vi "StartAndorCamera.vi"(2 "error in (no error)":errorcluster, 3 "Initial temp":i32) -> (0 "error out":errorcluster, 1 "Camera OK?":bool)   [LabVIEW 2019]
uses:
  <userlib>/atmcd32d.llb/Shutter_type typedef.ctl
  <userlib>/atmcd32d.llb/Shutter_mode typedef.ctl
panel:
  out "DLL error code":u32
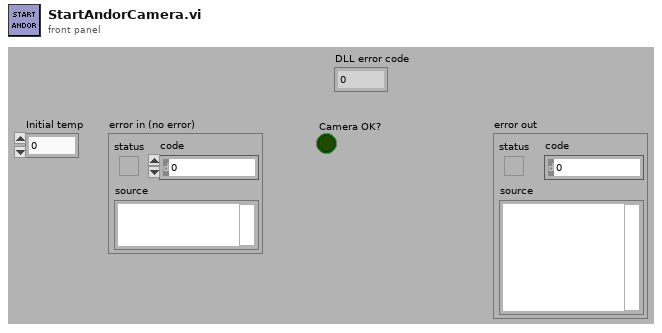
[diagram p1: front panel]
types:
  T1 = typedef "Shutter_mode typedef.ctl" = enum16{"Auto", "Open", "Close", "N/A (3)", "Open FVB Series", "Open Any Series"}
  T2 = typedef "Shutter_type typedef.ctl" = enum16{"TTL Low", "TTL High"}
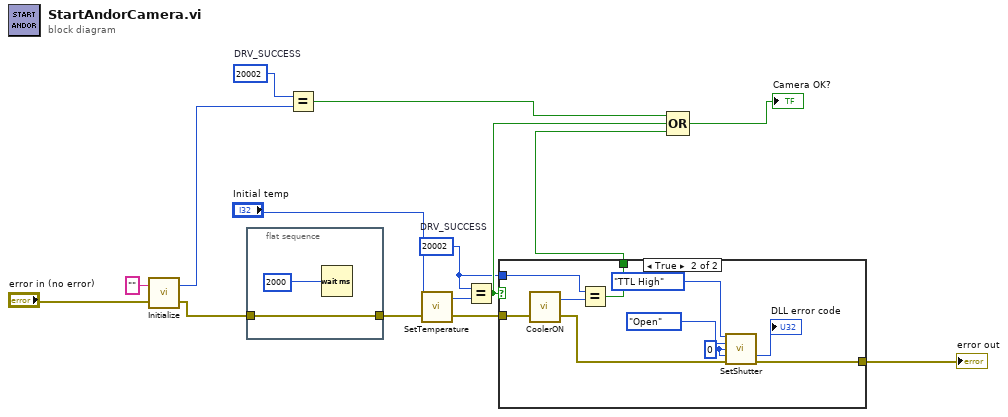
[diagram p0: block diagram]
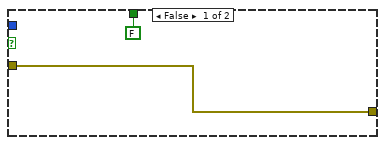
[diagram p2: hidden frame]
diagram:
  w12 = 20002  # DRV_SUCCESS
  w3 = 20002  # DRV_SUCCESS
  n1 = call <userlib>:"Initialize.vi"("error in (no error)"="error in (no error)", "directory (\"\")"="" ("directory (\"\")")) -> ("error out"=w11:errorcluster, "DLL error code"=w10:u32)
  n2 = flat-sequence {
    tunnel: w11 -> [w16]
    tunnel: [w16] -> w13
    frame #0 {
      n3 = Wait (ms)(milliseconds to wait=u32 2000) -> ()  [unwired: 1 out]
    }
  }
  n4 = Equal?(x=w12, y=w10) -> (x = y?=w5:bool)
  n5 = call <userlib>:"SetTemperature.vi"("error in (no error)"=w13, "temperature"="Initial temp") -> ("error out"=w8:errorcluster, "DLL error code"=w6:u32)
  n6 = Equal?(x=w3, y=w6) -> (x = y?=w4:bool)
  n7 = case shown="True" w4 {
    tunnel: w8 -> [w19 w29]
    tunnel: [w19 w22] -> w14
    tunnel: w3 -> [_ w27]
    tunnel: [FALSE w26] -> w2
    frame False {
    }
    frame True {
      w21 = 0 ("closingtime")
      n8 = call <userlib>:"CoolerON.vi"("error in (no error)"=w29) -> ("error out"=w23:errorcluster, "DLL error code"=w28:u32)  [unwired: 1 in]
      n9 = Equal?(x=w27, y=w28) -> (x = y?=w26:bool)
      n10 = call <userlib>:"SetShutter.vi"("type"=Shutter_type_typedef."TTL High", "mode"=Shutter_mode_typedef."Open", "closingtime"=w21, "openingtime"=w21, "error in (no error)"=w23) -> ("DLL error code"=→"DLL error code":u32, "error out"=w22:errorcluster)  [unwired: 9 in]
    }
  }
  "error out" <- w14
  n11 = Compound Arithmetic op=OR(w5, w4, w2) -> (→"Camera OK?":bool)
